vi "Loop.vi"(8 "error in (no error)":errorcluster, 11 "PID Loop in":refnum<class "PID Loop.lvclass">) -> (0 "error out":errorcluster, 3 "PID Loop out":refnum<class "PID Loop.lvclass">)   [LabVIEW 2024, in "PID Loop.lvlib" / "PID Loop.lvclass"]
uses:
  PID Loop.lvclass
  PID Loop.lvclass/PID Loop.ctl
  <vilib>/addons/control/pid/NI_PID_pid.lvlib
  <vilib>/addons/control/pid/pid.llb/PID (DBL).vi
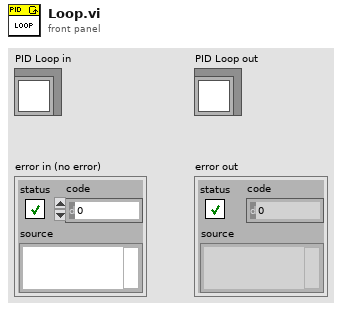
[diagram p1: front panel]
types:
  T1 = cluster{"proportional gain (Kc)":dbl, "integral time (Ti, min)":dbl, "derivative time (Td, min)":dbl}
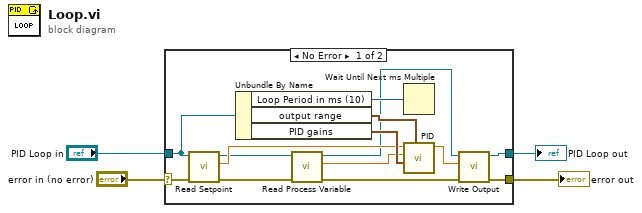
[diagram p0: block diagram]
diagram:
  n1 = case shown="No Error" "error in (no error)" {
    selector: "error in (no error)" -> [w15 w20]
    tunnel: [w8 w20] -> w3
    tunnel: [w7 w19] -> w1
    tunnel: "PID Loop in" -> [w5 w19]
    frame No Error {
      n2 = call-dynamic "Read Setpoint.vi"("error in (no error)"=w15, "PID Loop in"=w5) -> ("error out"=w12:errorcluster, "setpoint"=w14:dbl, "PID Loop out"=w13:refnum<class "PID Loop.lvclass">)  [unwired: 7 in]
      n3 = Unbundle By Name(w5) -> ("Loop Period in ms (10)"=w16:u32, "output range"=w18:cluster{"output high":dbl, "output low":dbl}, "PID gains"=w17:T1)
      n4 = call-dynamic "Read Process Variable.vi"("error in (no error)"=w12, "PID Loop in"=w13) -> ("error out"=w10:errorcluster, "process variable"=w11:dbl, "PID Loop out"=w6:refnum<class "PID Loop.lvclass">)  [unwired: 7 in]
      n5 = Wait Until Next ms Multiple(millisecond multiple=w16) -> ()  [unwired: 1 out]
      n6 = call-poly <vilib>:"PID.vi"("output range"=w18, "PID gains"=w17, "process variable"=w11, "setpoint"=w14) -> ("output"=w9:dbl)  [unwired: 6 in, 1 out]
      n7 = call-dynamic "Write Output.vi"("error in (no error)"=w10, "output"=w9, "PID Loop in"=w6) -> ("error out"=w8:errorcluster, "PID Loop out"=w7:refnum<class "PID Loop.lvclass">)  [unwired: 7 in]
    }
    frame Error {
    }
  }
  "error out" <- w3
  "PID Loop out" <- w1
